vi "M2p_AD_Std_ABA.vi"() -> ()   [LabVIEW 2015]
uses:
  spcm_library/spcm_gui_common.llb/element_device.ctl
  spcm_library/spcm_gui_common.llb/element_mode.ctl
  spcm_library/spcm_gui_m2p.llb/element_m2p_ai_channel.ctl
  spcm_library/spcm_gui_common.llb/element_device_infos.ctl
  spcm_library/spcm_gui_m2p.llb/element_m2p_clock.ctl
  spcm_library/spcm_gui_m2p.llb/element_m2p_ai_trigger.ctl
panel:
  in  "Trigger Settings":T1={"Trigger Source"=0, "External Trigger"=0, "Level 0 Ext"=1500, "Ext Trig Term"=FALSE, "Channel Trigger"=0, "Level 0 Ch"=0, "Level 1 Ch"=0, "Trigger Delay (Samples)"=0} {"Channel Trigger" items=["None", "Pos. Edge", "Neg. Edge", "Any Edge", "Pos. Rearm", "Neg. Rearm", "Enter Window", "Leave Window", "In Win", "Out Win"]; "External Trigger" items=["None", "Pos. Edge", "Neg. Edge", "Any Edge", "High Level", "Low Level"]; "Trigger Source" items=["Software Trigger", "External Trigger", "Channel 0 Trigger", "Channel 1 Trigger", "Channel 2 Trigger", "Channel 3 Trigger", "Channel 4 Trigger", "Channel 5 Trigger", "Channel 6 Trigger", "Channel 7 Trigger"]; "Trigger Delay (Samples)" max=65535 step=1}
  in  "Clock Settings":T2={"Clock Mode"=0, "Sampling Rate (kHz)"=10000.0, "Clock Output"=FALSE, "Termination"=FALSE, "Ref. Clock (MHz)"=10.0, "Threshold (mV)"=1500} {"Threshold (mV)" min=-5000 max=5000; "Clock Mode" items=["Internal Clock Quartz", "External Clock", "External Reference Clock"]; "Ref. Clock (MHz)" min=0.0 max=125000.0; "Sampling Rate (kHz)" min=1.0 max=5000000.0}
  out "Device Infos":T3={"Device Name"="M2p.5942-x4", "Serial Number"=666.0, "Mem (MB)"=1024.0}
  in  "AI Channel 7":T4={"Enable"=TRUE, "Input Range "=2, "Termination"=0, "Input Type"=0, "Offset"=0} {"Input Type" items=["Single-ended", "Differential"]; "Termination" items=["1 MOhm", "50 Ohm"]; "Input Range" items=["±200 mV", "±500 mV", "±1000 mV", "±2000 mV", "±5000 mV", "±10000 mV"]}
  in  "AI Channel 6":T4={"Enable"=TRUE, "Input Range "=2, "Termination"=0, "Input Type"=0, "Offset"=0} {"Input Type" items=["Single-ended", "Differential"]; "Termination" items=["1 MOhm", "50 Ohm"]; "Input Range" items=["±200 mV", "±500 mV", "±1000 mV", "±2000 mV", "±5000 mV", "±10000 mV"]}
  in  "AI Channel 5":T4={"Enable"=TRUE, "Input Range "=2, "Termination"=0, "Input Type"=0, "Offset"=0} {"Input Type" items=["Single-ended", "Differential"]; "Termination" items=["1 MOhm", "50 Ohm"]; "Input Range" items=["±200 mV", "±500 mV", "±1000 mV", "±2000 mV", "±5000 mV", "±10000 mV"]}
  in  "AI Channel 4":T4={"Enable"=TRUE, "Input Range "=2, "Termination"=0, "Input Type"=0, "Offset"=0} {"Input Type" items=["Single-ended", "Differential"]; "Termination" items=["1 MOhm", "50 Ohm"]; "Input Range" items=["±200 mV", "±500 mV", "±1000 mV", "±2000 mV", "±5000 mV", "±10000 mV"]}
  in  "AI Channel 3":T4={"Enable"=TRUE, "Input Range "=2, "Termination"=0, "Input Type"=0, "Offset"=0} {"Input Type" items=["Single-ended", "Differential"]; "Termination" items=["1 MOhm", "50 Ohm"]; "Input Range" items=["±200 mV", "±500 mV", "±1000 mV", "±2000 mV", "±5000 mV", "±10000 mV"]}
  in  "AI Channel 2":T4={"Enable"=TRUE, "Input Range "=2, "Termination"=0, "Input Type"=0, "Offset"=0} {"Input Type" items=["Single-ended", "Differential"]; "Termination" items=["1 MOhm", "50 Ohm"]; "Input Range" items=["±200 mV", "±500 mV", "±1000 mV", "±2000 mV", "±5000 mV", "±10000 mV"]}
  in  "AI Channel 1":T4={"Enable"=TRUE, "Input Range "=2, "Termination"=0, "Input Type"=0, "Offset"=0} {"Input Type" items=["Single-ended", "Differential"]; "Termination" items=["1 MOhm", "50 Ohm"]; "Input Range" items=["±200 mV", "±500 mV", "±1000 mV", "±2000 mV", "±5000 mV", "±10000 mV"]}
  in  "AI Channel 0":T4={"Enable"=TRUE, "Input Range "=2, "Termination"=0, "Input Type"=0, "Offset"=0} {"Input Type" items=["Single-ended", "Differential"]; "Termination" items=["1 MOhm", "50 Ohm"]; "Input Range" items=["±200 mV", "±500 mV", "±1000 mV", "±2000 mV", "±5000 mV", "±10000 mV"]}
  in  "Mode Setup":T5={"Mode"=3, "Mem"=16384, "Seg"=4096, "Post"=4000, "Pre"=32, "ABA"=1024} {"Mode" items=["Singleshot", "Multiple Recording", "Gated Sampling", "ABA Mode"]; "ABA" min=2 max=65535 step=1; "Post" min=4 step=4; "Mem" min=8 step=4; "Pre" min=4 max=8176 step=4; "Seg" min=8 step=4}
  in  "Loop Button":bool
  in  "Singleshot Button":bool
  in  "Quit Button":bool
  in  "Force Trigger Button":bool
  in  "Stop Button":bool
  out "Display ABA Data":sgl[][](graph)=[[-0.7367859, -0.9946289, -0.85287476, -0.3730774, 0.25793457, 0.7870178, 0.54119873, 0.93759155, 0.95895386, 0.5987854, -0.002960205, -0.6014404, -0.95977783, -0.9349365, -0.5342407, 0.078125, 0.6602783, 0.97946167, 0.9064636, 0.47125244, -0.15322876, -0.7137146, -0.9917908, -0.87109375, -0.40386963, 0.22634888, 0.76467896, 0.99749756, 0.8317261, 0.33291626, -0.29797363, -0.80978394, -0.9989319, -0.78674316, -0.262146, 0.36953735, 0.8530884, 0.99542236, 0.957428, 0.9367676, 0.95092773, 0.57244873, 0.9633179, 0.60528564, 0.6083679, 0.96325684, 0.9303894, 0.5276489, -0.08602905, -0.66571045, -0.9791565, -0.90148926, -0.4619751, 0.16055298, 0.7215271, 0.99157715, 0.8659668, 0.39404297, -0.23522949, -0.7704468, -0.9981079, -0.8261719, -0.32208252, 0.3079834, 0.8153076, 0.99713135, 0.7798767, 0.25057983, -0.3774109, -0.8551941, -0.9929199, -0.7310486, -0.17828369, 0.44638062, 0.8932495, 0.9847717, 0.6784668, 0.10494995, -0.51187134, -0.9230957, -0.9657898, -0.6234741, -0.028564453, 0.57696533, 0.9515686, 0.9458008, 0.56240845, -0.046081543, -0.63442993, -0.96972656, -0.9168701, -0.4967041, 0.122802734, 0.69241333, 0.9868469, 0.8860779, 0.43188477, -0.19503784, -0.7442627, -0.99487305, -0.84695435, -0.36273193, 0.26776123, 0.7922363, 0.999115, 0.8059082, 0.29092407, -0.33917236, -0.8347473, -0.99557495, -0.7579651, -0.21740723, 0.41140747, 0.87564087, 0.98968506, 0.70910645, 0.14578247, -0.47720337, -0.908844, -0.9749756, -0.6528015, -0.07043457, 0.5432129, 0.9382324, 0.9571533, 0.5940857, -0.0053100586, -0.60305786, -0.9604492, -0.9328613, -0.53204346, 0.081451416, 0.6625061, 0.9809265, 0.9046936, 0.46777344, -0.15338135, -0.7159729, -0.98999023, -0.86886597, -0.39935303, 0.22888184, 0.76641846, 0.99798584, 0.82928467, 0.32977295, -0.30187988, -0.8128662, -0.9975586, -0.7854004, -0.25775146, 0.37252808, 0.8534241, 0.9945984, 0.73779297, 0.18582153, -0.43966675, -0.88900757, -0.9826355, -0.6835327, -0.109191895, 0.50805664, 0.92178345, 0.96847534, 0.6272888, 0.03527832, -0.56951904, -0.9475403, -0.94628906, -0.56573486, 0.040740967, 0.63171387, 0.96813965, 0.9185791, 0.5029602, -0.11489868, -0.6854553, -0.9836731, -0.8875427, -0.4373169, 0.18899536, 0.7409973, 0.9963074, 0.85150146, 0.36868286, -0.26104736, -0.7892151, -0.99658203, -0.8095093, -0.2960205, 0.33428955, 0.8327942, 0.9961853, 0.76327515, 0.2255249, -0.40457153, -0.869751, -0.9884033, -0.71221924, -0.14993286, 0.47149658, 0.9060974, 0.9775696, 0.65753174, 0.077545166, -0.53515625, -0.9313965, -0.9560852, -0.60009766, -0.0017700195, 0.5982666, 0.9598999, 0.93588257, 0.5386658, -0.07458496, -0.65734863, -0.97714233, -0.9057312, -0.47232056, 0.14935303, 0.71273804, 0.9902649, 0.8724365, 0.40701294, -0.22207642, -0.7612915, -0.99557495, -0.8312683, -0.33428955, 0.2972412, 0.8088684, 0.9990845, 0.78948975, 0.26516724, -0.36514282, -0.8491211, -0.99346924, -0.7403259, -0.1906128, 0.4362793, 0.8887634, 0.9863281, 0.6897888, 0.11758423, -0.5010681, -0.9182129, -0.9694824, -0.6303711, -0.03970337, 0.56658936, 0.94696045, 0.9506836, 0.5725403, -0.032989502, -0.62384033, -0.96728516, -0.9217529, -0.50735474, 0.109802246, 0.6842346, 0.98431396, 0.89172363, 0.4421997, -0.18322754, -0.7343445, -0.99264526, -0.852478, -0.37271118, 0.25668335, 0.78564453, 0.99835205, 0.8143921, 0.3052063, -0.32714844, -0.82696533, -0.9963989, -0.7660217, -0.23092651, 0.3985901, 0.87039185, 0.99102783, 0.71658325, 0.15756226, -0.46670532, -0.9020996, -0.97735596, -0.6616821, -0.081970215, 0.53253174, 0.93270874, 0.96157837, 0.6053772, 0.0068359375, -0.59298706, -0.95565796, -0.936615, -0.5405884, 0.069732666, 0.65304565, 0.97595215, 0.9082947, 0.47894287, -0.14233398, -0.7063904, -0.9873657, -0.87454224, -0.41030884, 0.21688843, 0.7576294, 0.9977722, 0.8375244, 0.34188843, -0.2893982, -0.80496216, -0.99783325, -0.79125977, -0.2698059, 0.36218262, 0.8475952, 0.9964905, 0.7446289, 0.19586182, -0.42956543, -0.8841858, -0.9846802, -0.6915283, -0.12136841, 0.4963379, 0.9172058, 0.97128296, 0.63687134, 0.047454834, -0.56066895, -0.94454956, -0.94888306, -0.5776062, 0.029296875, 0.6207886, 0.9685974, 0.92419434, 0.5151367, -0.10394287, -0.67752075, -0.9823303, -0.8944092, -0.44708252, 0.17849731, 0.73184204, 0.9949646, 0.85809326, 0.3807068, -0.2501526, -0.7796631, -0.99731445, -0.8144226, -0.30908203, 0.32418823, 0.82598877, 0.9975891, 0.77267456, 0.23815918, -0.39318848, -0.86398315, -0.99017334, -0.72213745, -0.16357422, 0.4606018, 0.899353, 0.98202515, 0.6680908, 0.08944702, -0.5254822, -0.93099976, -0.9614258, -0.6101074, -0.013427734, 0.5890198, 0.9560852, 0.9404907, 0.5488281, -0.061035156, -0.6477356, -0.9737854, -0.91049194, -0.48309326, 0.13729858, 0.7044678, 0.9884033, 0.8786316, 0.41744995, -0.21096802, -0.7532959, -0.9957886, -0.8402405, -0.34680176, 0.28399658, 0.8029785, 0.999115, 0.7972717, 0.27694702, -0.35458374, -0.8433533, -0.9954834, -0.74780273, -0.20275879, 0.4248047, 0.88275146, 0.9875488, 0.69647217, 0.12808228, -0.49005127, -0.91326904, -0.9727478, -0.6412964, -0.052947998, 0.55615234, 0.9421997, 0.9526062, 0.58340454, -0.021606445, -0.6161804, -0.9637146, -0.9266052, -0.5185547, 0.097351074, 0.6750183, 0.98391724, 0.89624023, 0.45333862, -0.17086792, -0.727478, -0.9911194, -0.85980225, -0.38391113, 0.2453003, 0.7779846, 0.9977417, 0.8199463, 0.31497192, -0.31588745, -0.82162476, -0.9985962, -0.7744751, -0.24353027, 0.3881836, 0.8618164, 0.99365234, 0.7267761, 0.16906738, -0.45483398, -0.89715576, -0.9794922, -0.6708069, -0.094573975, 0.52267456, 0.9289856, 0.96435547, 0.61550903, 0.019927979, -0.5828247, -0.9527588, -0.94137573, -0.55200195, 0.057128906, 0.6442871, 0.97320557, 0.9138794, 0.48950195, -0.13064575, -0.69818115, -0.98669434, -0.88131714, -0.4220581, 0.20544434, 0.7498779, 0.9970703, 0.8441467, 0.35308838, -0.27630615, -0.7956543, -0.9975891, -0.7987366, -0.2817688, 0.3501892, 0.842926, 0.9965515, 0.75305176, 0.20935059, -0.41931152, -0.87841797, -0.9868164, -0.70007324, -0.13421631, 0.4862671, 0.9122009, 0.9748535, 0.6463318, 0.061462402, -0.5491638, -0.940155, -0.9536133, -0.58636475, 0.015380859, 0.61190796, 0.9640808, 0.9303589, 0.5248413, -0.089416504, -0.6679077, -0.9793701, -0.89849854, -0.45965576], [0.38497925, 0.38497925, 0.38497925, 0.38497925, 0.38497925, 0.38497925, 0.38497925, 0.38497925, 0.38497925, 0.38497925, 0.38497925, 0.38497925, 0.38497925, 0.38497925, 0.38497925, 0.38497925, 0.38497925, 0.38497925, 0.38497925, 0.38497925, 0.38497925, 0.38497925, 0.38497925, 0.38497925, 0.38497925, 0.38497925, 0.38497925, 0.38497925, 0.38497925, 0.38497925, 0.38497925, 0.38497925, 0.38497925, 0.38497925, 0.38497925, 0.38497925, 0.38497925, 0.38497925, 0.38497925, 0.38497925, 0.38497925, 0.38497925, 0.38497925, 0.38497925, 0.38497925, 0.38497925, 0.38497925, 0.38497925, 0.38497925, 0.38497925, 0.38497925, 0.38497925, 0.38497925, 0.38497925, 0.38497925, 0.38497925, 0.38497925, 0.38497925, 0.38497925, 0.38497925, 0.38497925, 0.38497925, 0.38497925, 0.38497925, 0.38497925, 0.38497925, 0.38497925, 0.38497925, 0.38497925, 0.38497925, 0.38497925, 0.38497925, 0.38497925, 0.38497925, 0.38497925, 0.38497925, 0.38497925, 0.38497925, 0.38497925, 0.38497925, 0.38497925, 0.38497925, 0.38497925, 0.38497925, 0.38497925, 0.38497925, 0.38497925, 0.38497925, 0.38497925, 0.38497925, 0.38497925, 0.38497925, 0.38497925, 0.38497925, 0.38497925, 0.38497925, 0.38497925, 0.38497925, 0.38497925, 0.38497925, 0.38497925, 0.38497925, 0.38497925, 0.38497925, 0.38497925, 0.38497925, 0.38497925, 0.38497925, 0.38497925, 0.38497925, 0.38497925, 0.38497925, 0.38497925, 0.38497925, 0.38497925, 0.38497925, 0.38497925, 0.38497925, 0.38497925, 0.38497925, 0.38497925, 0.38497925, 0.38497925, 0.38497925, 0.38497925, 0.38497925, 0.38497925, 0.38497925, 0.38497925, 0.38497925, 0.38497925, 0.38497925, 0.38497925, 0.38497925, 0.38497925, 0.38497925, 0.38497925, 0.38497925, 0.38497925, 0.38497925, 0.38497925, 0.38497925, 0.38497925, 0.38497925, 0.38497925, 0.38497925, 0.38497925, 0.38497925, 0.38497925, 0.38497925, 0.38497925, 0.38497925, 0.38497925, 0.38497925, 0.38497925, 0.38497925, 0.38497925, 0.38497925, 0.38497925, 0.38497925, 0.38497925, 0.38497925, 0.38497925, 0.38497925, 0.38497925, 0.38497925, 0.38497925, 0.38497925, 0.38497925, 0.38497925, 0.38497925, 0.38497925, 0.38497925, 0.38497925, 0.38497925, 0.38497925, 0.38497925, 0.38497925, 0.38497925, 0.38497925, 0.38497925, 0.38497925, 0.38497925, 0.38497925, 0.38497925, 0.38497925, 0.38497925, 0.38497925, 0.38497925, 0.38497925, 0.38497925, 0.38497925, 0.38497925, 0.38497925, 0.38497925, 0.38497925, 0.38497925, 0.38497925, 0.38497925, 0.38497925, 0.38497925, 0.38497925, 0.38497925, 0.38497925, 0.38497925, 0.38497925, 0.38497925, 0.38497925, 0.38497925, 0.38497925, 0.38497925, 0.38497925, 0.38497925, 0.38497925, 0.38497925, 0.38497925, 0.38497925, 0.38497925, 0.38497925, 0.38497925, 0.38497925, 0.38497925, 0.38497925, 0.38497925, 0.38497925, 0.38497925, 0.38497925, 0.38497925, 0.38497925, 0.38497925, 0.38497925, 0.38497925, 0.38497925, 0.38497925, 0.38497925, 0.38497925, 0.38497925, 0.38497925, 0.38497925, 0.38497925, 0.38497925, 0.38497925, 0.38497925, 0.38497925, 0.38497925, 0.38497925, 0.38497925, 0.38497925, 0.38497925, 0.38497925, 0.38497925, 0.38497925, 0.38497925, 0.38497925, 0.38497925, 0.38497925, 0.38497925, 0.38497925, 0.38497925, 0.38497925, 0.38497925, 0.38497925, 0.38497925, 0.38497925, 0.38497925, 0.38497925, 0.38497925, 0.38497925, 0.38497925, 0.38497925, 0.38497925, 0.38497925, 0.38497925, 0.38497925, 0.38497925, 0.38497925, 0.38497925, 0.38497925, 0.38497925, 0.38497925, 0.38497925, 0.38497925, 0.38497925, 0.38497925, 0.38497925, 0.38497925, 0.38497925, 0.38497925, 0.38497925, 0.38497925, 0.38497925, 0.38497925, 0.38497925, 0.38497925, 0.38497925, 0.38497925, 0.38497925, 0.38497925, 0.38497925, 0.38497925, 0.38497925, 0.38497925, 0.38497925, 0.38497925, 0.38497925, 0.38497925, 0.38497925, 0.38497925, 0.38497925, 0.38497925, 0.38497925, 0.38497925, 0.38497925, 0.38497925, 0.38497925, 0.38497925, 0.38497925, 0.38497925, 0.38497925, 0.38497925, 0.38497925, 0.38497925, 0.38497925, 0.38497925, 0.38497925, 0.38497925, 0.38497925, 0.38497925, 0.38497925, 0.38497925, 0.38497925, 0.38497925, 0.38497925, 0.38497925, 0.38497925, 0.38497925, 0.38497925, 0.38497925, 0.38497925, 0.38497925, 0.38497925, 0.38497925, 0.38497925, 0.38497925, 0.38497925, 0.38497925, 0.38497925, 0.38497925, 0.38497925, 0.38497925, 0.38497925, 0.38497925, 0.38497925, 0.38497925, 0.38497925, 0.38497925, 0.38497925, 0.38497925, 0.38497925, 0.38497925, 0.38497925, 0.38497925, 0.38497925, 0.38497925, 0.38497925, 0.38497925, 0.38497925, 0.38497925, 0.38497925, 0.38497925, 0.38497925, 0.38497925, 0.38497925, 0.38497925, 0.38497925, 0.38497925, 0.38497925, 0.38497925, 0.38497925, 0.38497925, 0.38497925, 0.38497925, 0.38497925, 0.38497925, 0.38497925, 0.38497925, 0.38497925, 0.38497925, 0.38497925, 0.38497925, 0.38497925, 0.38497925, 0.38497925, 0.38497925, 0.38497925, 0.38497925, 0.38497925, 0.38497925, 0.38497925, 0.38497925, 0.38497925, 0.38497925, 0.38497925, 0.38497925, 0.38497925, 0.38497925, 0.38497925, 0.38497925, 0.38497925, 0.38497925, 0.38497925, 0.38497925, 0.38497925, 0.38497925, 0.38497925, 0.38497925, 0.38497925, 0.38497925, 0.38497925, 0.38497925, 0.38497925, 0.38497925, 0.38497925, 0.38497925, 0.38497925, 0.38497925, 0.38497925, 0.38497925, 0.38497925, 0.38497925, 0.38497925, 0.38497925, 0.38497925, 0.38497925, 0.38497925, 0.38497925, 0.38497925, 0.38497925, 0.38497925, 0.38497925, 0.38497925, 0.38497925, 0.38497925, 0.38497925, 0.38497925, 0.38497925, 0.38497925, 0.38497925, 0.38497925, 0.38497925, 0.38497925, 0.38497925, 0.38497925, 0.38497925, 0.38497925, 0.38497925, 0.38497925, 0.38497925, 0.38497925, 0.38497925, 0.38497925, 0.38497925, 0.38497925, 0.38497925, 0.38497925, 0.38497925, 0.38497925, 0.38497925, 0.38497925, 0.38497925, 0.38497925, 0.38497925, 0.38497925, 0.38497925, 0.38497925, 0.38497925, 0.38497925, 0.38497925, 0.38497925, 0.38497925, 0.38497925, 0.38497925, 0.38497925, 0.38497925, 0.38497925, 0.38497925, 0.38497925, 0.38497925, 0.38497925, 0.38497925, 0.38497925, 0.38497925, 0.38497925, 0.38497925, 0.38497925, 0.38497925, 0.38497925, 0.38497925, 0.38497925, 0.38497925, 0.38497925, 0.38497925, 0.38497925, 0.38497925, 0.38497925, 0.38497925, 0.38497925, 0.38497925, 0.38497925, 0.38497925, 0.38497925, 0.38497925], [-0.00012207031, -0.00012207031, -6.1035156e-05, -0.00012207031, 0.00015258789, -9.1552734e-05, 0.0, 0.00015258789, -0.00018310547, -6.1035156e-05, -0.00012207031, -3.0517578e-05, 0.00015258789, -0.00012207031, 6.1035156e-05, -3.0517578e-05, -6.1035156e-05, -0.00012207031, -0.00015258789, 0.00012207031, 6.1035156e-05, 3.0517578e-05, 3.0517578e-05, -6.1035156e-05, -0.00012207031, 0.0, 0.0, -6.1035156e-05, -9.1552734e-05, -0.00030517578, 0.0, 0.00015258789, 0.00015258789, -0.00030517578, -0.00015258789, 3.0517578e-05, 0.00018310547, -0.00018310547, -6.1035156e-05, -0.00012207031, -0.00012207031, -9.1552734e-05, -0.00015258789, -6.1035156e-05, -3.0517578e-05, -6.1035156e-05, -6.1035156e-05, -0.0002746582, 0.0, -6.1035156e-05, 3.0517578e-05, 9.1552734e-05, -0.00012207031, 3.0517578e-05, -9.1552734e-05, -9.1552734e-05, 0.00012207031, -3.0517578e-05, -0.00021362305, -6.1035156e-05, 3.0517578e-05, -3.0517578e-05, -6.1035156e-05, 0.0, -9.1552734e-05, 0.00012207031, -0.00018310547, -6.1035156e-05, 3.0517578e-05, 0.00012207031, 0.0002746582, 0.0, -0.00030517578, -0.00039672852, -0.00018310547, 3.0517578e-05, -0.00015258789, 0.00012207031, -0.00012207031, 0.00015258789, 6.1035156e-05, -0.00018310547, -0.00012207031, 0.00015258789, -0.00015258789, 3.0517578e-05, -6.1035156e-05, -0.00012207031, 0.0, 3.0517578e-05, 9.1552734e-05, -3.0517578e-05, -0.00021362305, 6.1035156e-05, -0.00012207031, -0.00018310547, 0.0, 6.1035156e-05, -9.1552734e-05, -0.00018310547, 0.0, -0.00015258789, -0.00021362305, -0.00018310547, 0.00012207031, 6.1035156e-05, 6.1035156e-05, -9.1552734e-05, -6.1035156e-05, -9.1552734e-05, -0.00012207031, 0.00015258789, 6.1035156e-05, 6.1035156e-05, 0.00018310547, -0.00030517578, -3.0517578e-05, 0.00012207031, -9.1552734e-05, -6.1035156e-05, 0.0, -6.1035156e-05, 0.0, -6.1035156e-05, -0.00012207031, 6.1035156e-05, 0.00015258789, 0.00021362305, -0.00015258789, -0.00012207031, -0.00012207031, -0.00012207031, 0.0, -3.0517578e-05, -0.00012207031, 0.0, -6.1035156e-05, 0.00015258789, 0.0, 0.0, 0.0, -9.1552734e-05, 6.1035156e-05, -9.1552734e-05, -3.0517578e-05, 6.1035156e-05, 3.0517578e-05, 3.0517578e-05, -0.00018310547, -0.00018310547, 6.1035156e-05, 0.0, -0.00018310547, -0.0002746582, 0.00012207031, 0.00012207031, -0.0002746582, 9.1552734e-05, 0.0, 9.1552734e-05, -0.00015258789, 6.1035156e-05, -0.0002746582, 0.0, 0.00024414062, 6.1035156e-05, -0.00021362305, -0.00015258789, -0.00021362305, 3.0517578e-05, 0.0, -0.00015258789, 6.1035156e-05, -3.0517578e-05, 0.0, 0.0, 3.0517578e-05, 6.1035156e-05, -0.00018310547, 0.00015258789, 6.1035156e-05, -3.0517578e-05, 3.0517578e-05, -3.0517578e-05, 0.00012207031, 0.00024414062, -6.1035156e-05, -0.00015258789, 0.0, 0.0, -0.00021362305, 9.1552734e-05, -0.00018310547, 6.1035156e-05, 6.1035156e-05, 9.1552734e-05, -6.1035156e-05, -0.00021362305, -0.00021362305, -0.00012207031, -9.1552734e-05, -0.0005187988, 0.00012207031, 0.0, 0.00018310547, 0.0, 0.00018310547, -3.0517578e-05, 0.0, 0.0, -0.00012207031, -6.1035156e-05, -3.0517578e-05, -9.1552734e-05, 9.1552734e-05, -6.1035156e-05, 0.0, 0.00012207031, -3.0517578e-05, -9.1552734e-05, 6.1035156e-05, -0.00018310547, -0.00024414062, -0.00018310547, -6.1035156e-05, -3.0517578e-05, 0.0, 3.0517578e-05, 6.1035156e-05, -9.1552734e-05, -6.1035156e-05, -0.00021362305, 3.0517578e-05, -0.00012207031, 6.1035156e-05, -0.00012207031, 3.0517578e-05, 0.00018310547, 3.0517578e-05, -9.1552734e-05, -9.1552734e-05, -0.00018310547, 0.0, -3.0517578e-05, -6.1035156e-05, -0.00012207031, 9.1552734e-05, 0.0, -0.00012207031, -3.0517578e-05, 3.0517578e-05, 0.00015258789, 0.00021362305, -0.00048828125, -3.0517578e-05, -6.1035156e-05, -0.00012207031, -9.1552734e-05, -6.1035156e-05, -0.00015258789, 0.0, -0.00012207031, 0.00018310547, 0.00012207031, 0.0, 3.0517578e-05, -6.1035156e-05, 9.1552734e-05, 0.00012207031, 6.1035156e-05, -0.00012207031, 6.1035156e-05, 3.0517578e-05, 0.00021362305, -0.00015258789, -6.1035156e-05, 6.1035156e-05, 3.0517578e-05, 0.0, 3.0517578e-05, -3.0517578e-05, 6.1035156e-05, 6.1035156e-05, 0.00012207031, 0.0, 9.1552734e-05, 3.0517578e-05, -0.00018310547, -0.00012207031, 6.1035156e-05, 0.0, -6.1035156e-05, 9.1552734e-05, -6.1035156e-05, 0.0, -6.1035156e-05, 0.0, -9.1552734e-05, 3.0517578e-05, 6.1035156e-05, -6.1035156e-05, -0.00015258789, -0.00012207031, 0.0, -9.1552734e-05, -0.00018310547, -6.1035156e-05, -0.00012207031, 3.0517578e-05, 0.00018310547, -0.00012207031, 9.1552734e-05, 0.00015258789, 0.00018310547, -0.00015258789, 6.1035156e-05, -0.00024414062, -0.00012207031, 0.00015258789, -0.00021362305, 0.0, 0.0, 0.00024414062, 6.1035156e-05, 0.0, 3.0517578e-05, 0.0, -0.00015258789, -9.1552734e-05, 0.00012207031, -3.0517578e-05, 6.1035156e-05, -0.00021362305, -9.1552734e-05, -3.0517578e-05, 6.1035156e-05, -0.00015258789, -6.1035156e-05, -0.00021362305, -3.0517578e-05, 9.1552734e-05, -3.0517578e-05, -0.00015258789, 0.0, 0.0, 0.0, -9.1552734e-05, 0.00012207031, -0.00018310547, -0.00024414062, -0.00021362305, 0.00012207031, -0.00015258789, -9.1552734e-05, -0.00024414062, -3.0517578e-05, 0.0, 0.00033569336, 0.0, -0.00021362305, 9.1552734e-05, -6.1035156e-05, -0.00021362305, -3.0517578e-05, -0.00012207031, -9.1552734e-05, -0.00036621094, -0.0002746582, -0.00015258789, 6.1035156e-05, -3.0517578e-05, 0.00030517578, 0.0, -0.00012207031, 0.00018310547, -3.0517578e-05, -0.00015258789, -6.1035156e-05, 6.1035156e-05, 0.0, 9.1552734e-05, -0.00015258789, -6.1035156e-05, -0.00015258789, -3.0517578e-05, 0.0, -0.00021362305, -6.1035156e-05, -9.1552734e-05, -3.0517578e-05, 3.0517578e-05, -0.00012207031, -0.0002746582, -3.0517578e-05, 0.00012207031, -0.00012207031, -0.00012207031, -0.00030517578, -0.00021362305, 3.0517578e-05, 0.00012207031, 0.0, 3.0517578e-05, 6.1035156e-05, -9.1552734e-05, -3.0517578e-05, 0.00015258789, 0.00012207031, 3.0517578e-05, 3.0517578e-05, -6.1035156e-05, -0.00015258789, -3.0517578e-05, -3.0517578e-05, -9.1552734e-05, -3.0517578e-05, -6.1035156e-05, -0.00012207031, 0.0, -0.00018310547, 3.0517578e-05, -6.1035156e-05, 0.0, 3.0517578e-05, -3.0517578e-05, -3.0517578e-05, -0.00012207031, 0.0, 6.1035156e-05, -9.1552734e-05, 6.1035156e-05, -0.00015258789, -0.00021362305, -0.00021362305, 3.0517578e-05, -3.0517578e-05, -3.0517578e-05, 6.1035156e-05, -9.1552734e-05, 0.0, -9.1552734e-05, 3.0517578e-05, -0.00015258789, -9.1552734e-05, -3.0517578e-05, -3.0517578e-05, -6.1035156e-05, 0.00015258789, -6.1035156e-05, -0.00021362305, -3.0517578e-05, 9.1552734e-05, -0.00024414062, -3.0517578e-05, -6.1035156e-05, -0.00024414062, 0.0, 9.1552734e-05, -0.00015258789, 6.1035156e-05, -0.00012207031, 0.0, -6.1035156e-05, -0.00012207031, -3.0517578e-05, 0.0, -9.1552734e-05, 9.1552734e-05, -0.00012207031, 9.1552734e-05, -0.0002746582, -0.00012207031, 0.0, 0.00012207031, -3.0517578e-05, 0.0, 0.0, -9.1552734e-05, 9.1552734e-05, -9.1552734e-05, -0.00015258789, 0.0, -0.00018310547, 0.0, -6.1035156e-05, -3.0517578e-05, -3.0517578e-05, 6.1035156e-05, -9.1552734e-05, 9.1552734e-05, -9.1552734e-05, 0.00015258789, -0.00033569336, -3.0517578e-05, 6.1035156e-05, 0.00015258789, 3.0517578e-05, -0.00015258789, 0.00012207031, 9.1552734e-05, 0.0, -9.1552734e-05, -0.00012207031, 0.0, 3.0517578e-05, -9.1552734e-05, -6.1035156e-05, -0.00018310547, -3.0517578e-05, -0.00021362305, 9.1552734e-05, -9.1552734e-05], [0.1260376, 0.1260376, 0.1260376, 0.1260376, 0.1260376, 0.1260376, 0.1260376, 0.1260376, 0.1260376, 0.1260376, 0.1260376, 0.1260376, 0.1260376, 0.1260376, 0.1260376, 0.1260376, 0.1260376, 0.1260376, 0.1260376, 0.1260376, 0.1260376, 0.1260376, 0.1260376, 0.1260376, 0.1260376, 0.1260376, 0.1260376, 0.1260376, 0.1260376, 0.1260376, 0.1260376, 0.1260376, 0.1260376, 0.1260376, 0.1260376, 0.1260376, 0.1260376, 0.1260376, 0.1260376, 0.1260376, 0.1260376, 0.1260376, 0.1260376, 0.1260376, 0.1260376, 0.1260376, 0.1260376, 0.1260376, 0.1260376, 0.1260376, 0.1260376, 0.1260376, 0.1260376, 0.1260376, 0.1260376, 0.1260376, 0.1260376, 0.1260376, 0.1260376, 0.1260376, 0.1260376, 0.1260376, 0.1260376, 0.1260376, 0.1260376, 0.1260376, 0.1260376, 0.1260376, 0.1260376, 0.1260376, 0.1260376, 0.1260376, 0.1260376, 0.1260376, 0.1260376, 0.1260376, 0.1260376, 0.1260376, 0.1260376, 0.1260376, 0.1260376, 0.1260376, 0.1260376, 0.1260376, 0.1260376, 0.1260376, 0.1260376, 0.1260376, 0.1260376, 0.1260376, 0.1260376, 0.1260376, 0.1260376, 0.1260376, 0.1260376, 0.1260376, 0.1260376, 0.1260376, 0.1260376, 0.1260376, 0.1260376, 0.1260376, 0.1260376, 0.1260376, 0.1260376, 0.1260376, 0.1260376, 0.1260376, 0.1260376, 0.1260376, 0.1260376, 0.1260376, 0.1260376, 0.1260376, 0.1260376, 0.1260376, 0.1260376, 0.1260376, 0.1260376, 0.1260376, 0.1260376, 0.1260376, 0.1260376, 0.1260376, 0.1260376, 0.1260376, 0.1260376, 0.1260376, 0.1260376, 0.1260376, 0.1260376, 0.1260376, 0.1260376, 0.1260376, 0.1260376, 0.1260376, 0.1260376, 0.1260376, 0.1260376, 0.1260376, 0.1260376, 0.1260376, 0.1260376, 0.1260376, 0.1260376, 0.1260376, 0.1260376, 0.1260376, 0.1260376, 0.1260376, 0.1260376, 0.1260376, 0.1260376, 0.1260376, 0.1260376, 0.1260376, 0.1260376, 0.1260376, 0.1260376, 0.1260376, 0.1260376, 0.1260376, 0.1260376, 0.1260376, 0.1260376, 0.1260376, 0.1260376, 0.1260376, 0.1260376, 0.1260376, 0.1260376, 0.1260376, 0.1260376, 0.1260376, 0.1260376, 0.1260376, 0.1260376, 0.1260376, 0.1260376, 0.1260376, 0.1260376, 0.1260376, 0.1260376, 0.1260376, 0.1260376, 0.1260376, 0.1260376, 0.1260376, 0.1260376, 0.1260376, 0.1260376, 0.1260376, 0.1260376, 0.1260376, 0.1260376, 0.1260376, 0.1260376, 0.1260376, 0.1260376, 0.1260376, 0.1260376, 0.1260376, 0.1260376, 0.1260376, 0.1260376, 0.1260376, 0.1260376, 0.1260376, 0.1260376, 0.1260376, 0.1260376, 0.1260376, 0.1260376, 0.1260376, 0.1260376, 0.1260376, 0.1260376, 0.1260376, 0.1260376, 0.1260376, 0.1260376, 0.1260376, 0.1260376, 0.1260376, 0.1260376, 0.1260376, 0.1260376, 0.1260376, 0.1260376, 0.1260376, 0.1260376, 0.1260376, 0.1260376, 0.1260376, 0.1260376, 0.1260376, 0.1260376, 0.1260376, 0.1260376, 0.1260376, 0.1260376, 0.1260376, 0.1260376, 0.1260376, 0.1260376, 0.1260376, 0.1260376, 0.1260376, 0.1260376, 0.1260376, 0.1260376, 0.1260376, 0.1260376, 0.1260376, 0.1260376, 0.1260376, 0.1260376, 0.1260376, 0.1260376, 0.1260376, 0.1260376, 0.1260376, 0.1260376, 0.1260376, 0.1260376, 0.1260376, 0.1260376, 0.1260376, 0.1260376, 0.1260376, 0.1260376, 0.1260376, 0.1260376, 0.1260376, 0.1260376, 0.1260376, 0.1260376, 0.1260376, 0.1260376, 0.1260376, 0.1260376, 0.1260376, 0.1260376, 0.1260376, 0.1260376, 0.1260376, 0.1260376, 0.1260376, 0.1260376, 0.1260376, 0.1260376, 0.1260376, 0.1260376, 0.1260376, 0.1260376, 0.1260376, 0.1260376, 0.1260376, 0.1260376, 0.1260376, 0.1260376, 0.1260376, 0.1260376, 0.1260376, 0.1260376, 0.1260376, 0.1260376, 0.1260376, 0.1260376, 0.1260376, 0.1260376, 0.1260376, 0.1260376, 0.1260376, 0.1260376, 0.1260376, 0.1260376, 0.1260376, 0.1260376, 0.1260376, 0.1260376, 0.1260376, 0.1260376, 0.1260376, 0.1260376, 0.1260376, 0.1260376, 0.1260376, 0.1260376, 0.1260376, 0.1260376, 0.1260376, 0.1260376, 0.1260376, 0.1260376, 0.1260376, 0.1260376, 0.1260376, 0.1260376, 0.1260376, 0.1260376, 0.1260376, 0.1260376, 0.1260376, 0.1260376, 0.1260376, 0.1260376, 0.1260376, 0.1260376, 0.1260376, 0.1260376, 0.1260376, 0.1260376, 0.1260376, 0.1260376, 0.1260376, 0.1260376, 0.1260376, 0.1260376, 0.1260376, 0.1260376, 0.1260376, 0.1260376, 0.1260376, 0.1260376, 0.1260376, 0.1260376, 0.1260376, 0.1260376, 0.1260376, 0.1260376, 0.1260376, 0.1260376, 0.1260376, 0.1260376, 0.1260376, 0.1260376, 0.1260376, 0.1260376, 0.1260376, 0.1260376, 0.1260376, 0.1260376, 0.1260376, 0.1260376, 0.1260376, 0.1260376, 0.1260376, 0.1260376, 0.1260376, 0.1260376, 0.1260376, 0.1260376, 0.1260376, 0.1260376, 0.1260376, 0.1260376, 0.1260376, 0.1260376, 0.1260376, 0.1260376, 0.1260376, 0.1260376, 0.1260376, 0.1260376, 0.1260376, 0.1260376, 0.1260376, 0.1260376, 0.1260376, 0.1260376, 0.1260376, 0.1260376, 0.1260376, 0.1260376, 0.1260376, 0.1260376, 0.1260376, 0.1260376, 0.1260376, 0.1260376, 0.1260376, 0.1260376, 0.1260376, 0.1260376, 0.1260376, 0.1260376, 0.1260376, 0.1260376, 0.1260376, 0.1260376, 0.1260376, 0.1260376, 0.1260376, 0.1260376, 0.1260376, 0.1260376, 0.1260376, 0.1260376, 0.1260376, 0.1260376, 0.1260376, 0.1260376, 0.1260376, 0.1260376, 0.1260376, 0.1260376, 0.1260376, 0.1260376, 0.1260376, 0.1260376, 0.1260376, 0.1260376, 0.1260376, 0.1260376, 0.1260376, 0.1260376, 0.1260376, 0.1260376, 0.1260376, 0.1260376, 0.1260376, 0.1260376, 0.1260376, 0.1260376, 0.1260376, 0.1260376, 0.1260376, 0.1260376, 0.1260376, 0.1260376, 0.1260376, 0.1260376, 0.1260376, 0.1260376, 0.1260376, 0.1260376, 0.1260376, 0.1260376, 0.1260376, 0.1260376, 0.1260376, 0.1260376, 0.1260376, 0.1260376, 0.1260376, 0.1260376, 0.1260376, 0.1260376, 0.1260376, 0.1260376, 0.1260376, 0.1260376, 0.1260376, 0.1260376, 0.1260376, 0.1260376, 0.1260376, 0.1260376, 0.1260376, 0.1260376, 0.1260376, 0.1260376, 0.1260376, 0.1260376, 0.1260376, 0.1260376, 0.1260376, 0.1260376, 0.1260376, 0.1260376, 0.1260376]]
  out "Write Setup":bool
  out "Status":string="Stopped"
  out "Display Data":sgl[][](graph)
  in  "Device":T6 {"Device" items=["Card", "digitizerNETBOX"]}
  # "M2p ABA Example"
  # "Mode Settings"
  # "Range"
  # "Term"
  # "Type"
  # "Offset"
  # "Ch0"
  # "Ch1"
  # "Clock Settings"
  # "Ch2"
  # "Ch3"
  # "Ch4"
  # "Trigger Settings"
  # "Ch5"
  # "Ch6"
  # "Ch7"
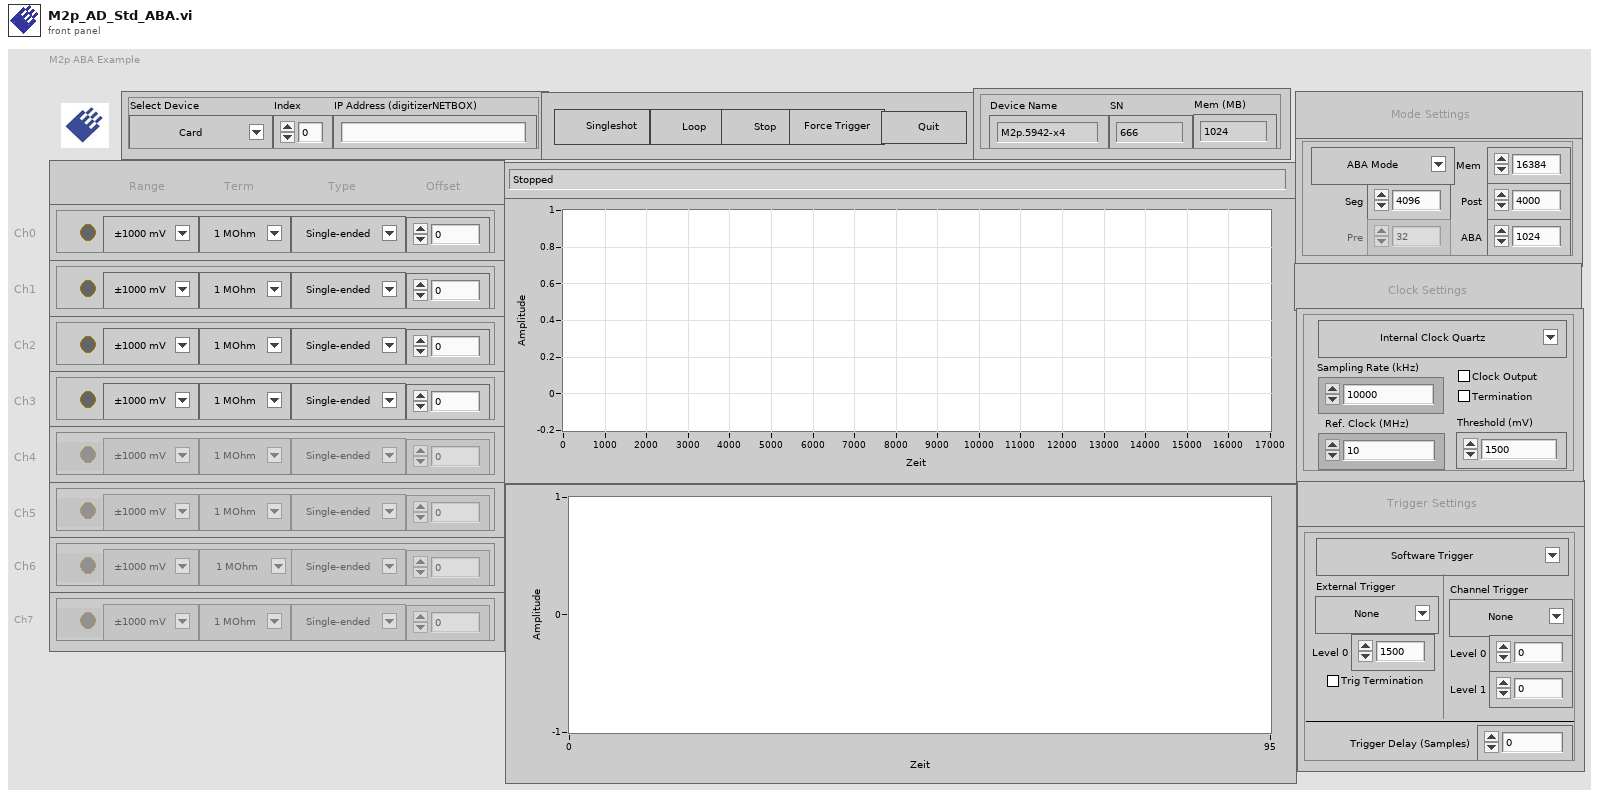
[diagram p1: front panel]
types:
  T1 = typedef "element_m2p_ai_trigger.ctl" = cluster{"Trigger Source":u16, "External Trigger":u16, "Level 0 Ext":i32, "Ext Trig Term":bool, "Channel Trigger":u16, "Level 0 Ch":i32, "Level 1 Ch":i32, "Trigger Delay (Samples)":u32}
  T2 = typedef "element_m2p_clock.ctl" = cluster{"Clock Mode":u16, "Sampling Rate (kHz)":dbl, "Clock Output":bool, "Termination":bool, "Ref. Clock (MHz)":dbl, "Threshold (mV)":i32}
  T3 = typedef "element_device_infos.ctl" = cluster{"Device Name":string, "Serial Number":dbl, "Mem (MB)":dbl}
  T4 = typedef "element_m2p_ai_channel.ctl" = cluster{"Enable":bool, "Input Range ":u16, "Termination":u16, "Input Type":u16, "Offset":i32}
  T5 = typedef "element_mode.ctl" = cluster{"Mode":u16, "Mem":u32, "Seg":u32, "Post":u32, "Pre":u32, "ABA":u32}
  T6 = typedef "element_device.ctl" = cluster{"Index":dbl, "IP Address":string, "Device":u16}
  T7 = enum16{"Idle", "Init", "Write Setup", "Start", "Acquire", "Read Data", "Stop", "Quit"}
  T8 = cluster{"Card Type":i32, "Inst Mem (high part)":i32, "Inst Mem (low part)":i32, "Serial Number":i32, "Function Type":i32, "Installed Features":i32, "Base Card Version":i32, "Module Version":i32, "Extension Version":i32, "Production Date":i32, "Max Sampling Rate":i32, "Max Channels":i32, "Demo Card":i32}
  T9 = cluster{"Card Name":string, "SN":i32, "Mem (MB)":i32}
  T10 = cluster{"AI Channels":i32, "AI Ranges":i32, "Input Ranges (mV)":i32[], "Programmable Offset":i32, "Termination Available":bool, "SE/Diff switchable":bool, "Offset in per cent/mV":bool, "Offset Calibration":bool, "Gain Calibration":bool, "Offset with open inputs":bool, "AI Range Strings[]":string[], "Bit Resolution":i32, "AC Coupling available":bool, "BW Limit available":bool, "AI Path count":i32}
  T11 = enum16{"Idle", "Init", "Write Setup", "Start", "Acquire", "Read Data", "Quit"}
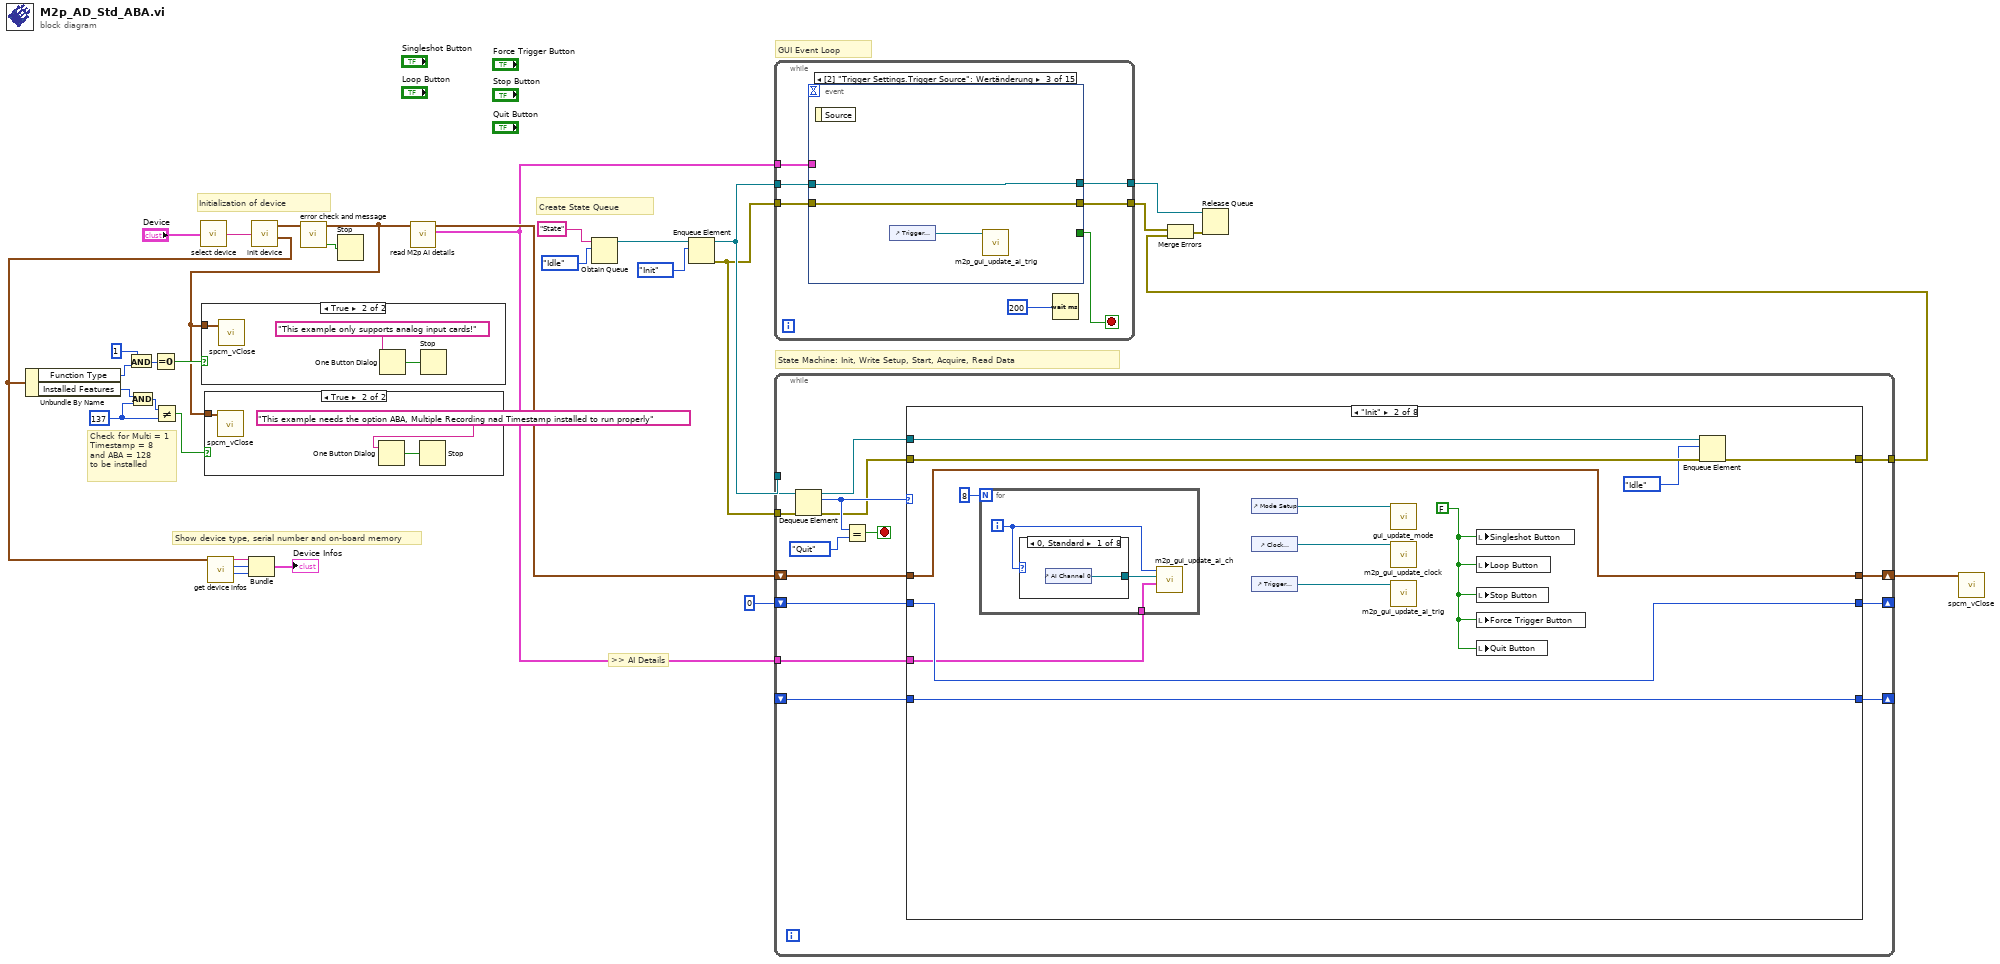
[diagram p0: block diagram]
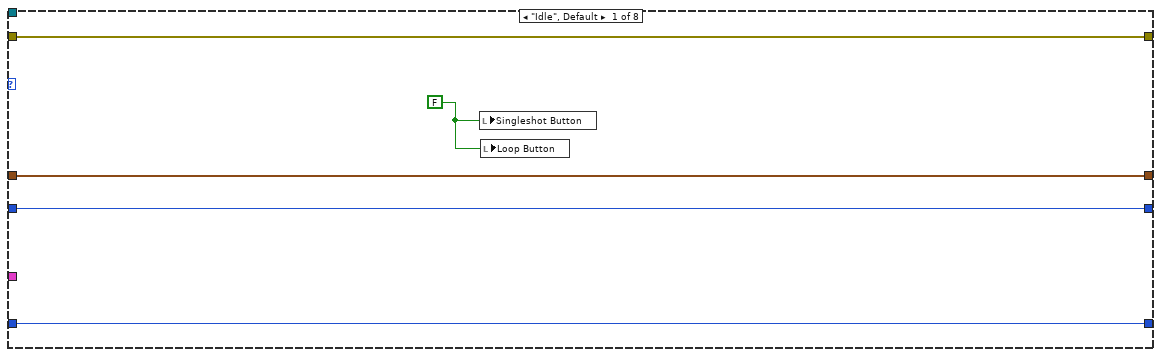
[diagram p4: hidden frame]
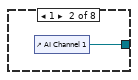
[diagram p5: hidden frame]
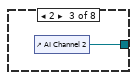
[diagram p6: hidden frame]
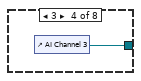
[diagram p7: hidden frame]
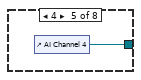
[diagram p8: hidden frame]
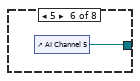
[diagram p9: hidden frame]
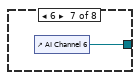
[diagram p10: hidden frame]
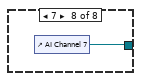
[diagram p11: hidden frame]
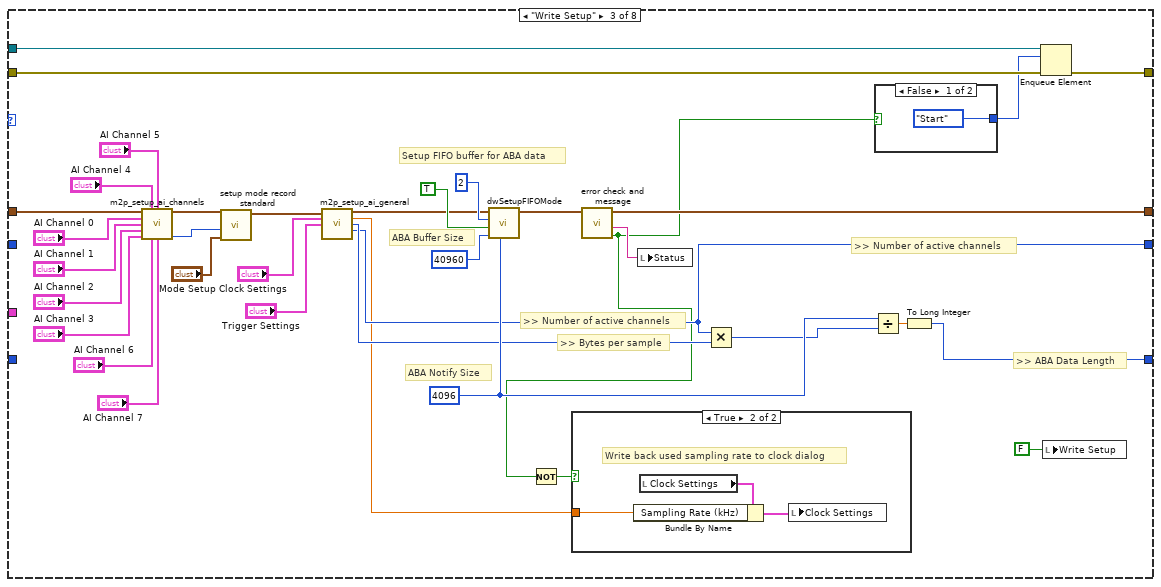
[diagram p12: hidden frame]
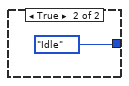
[diagram p14: hidden frame]
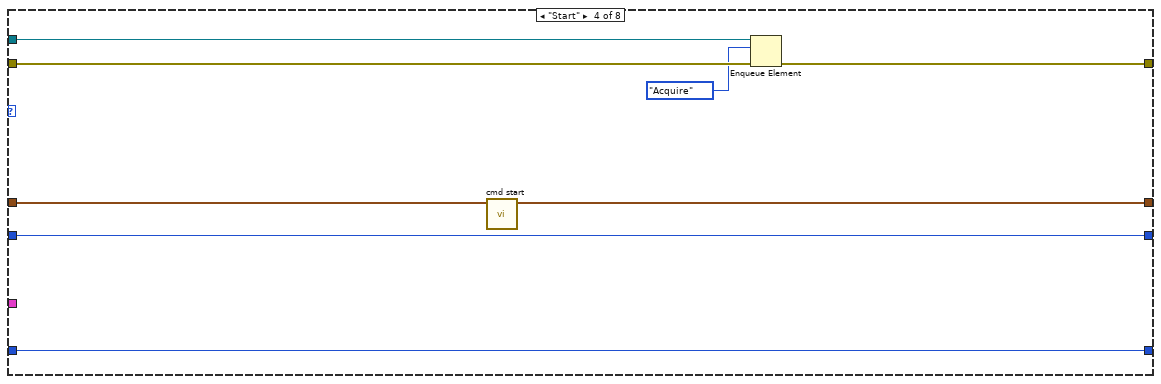
[diagram p15: hidden frame]
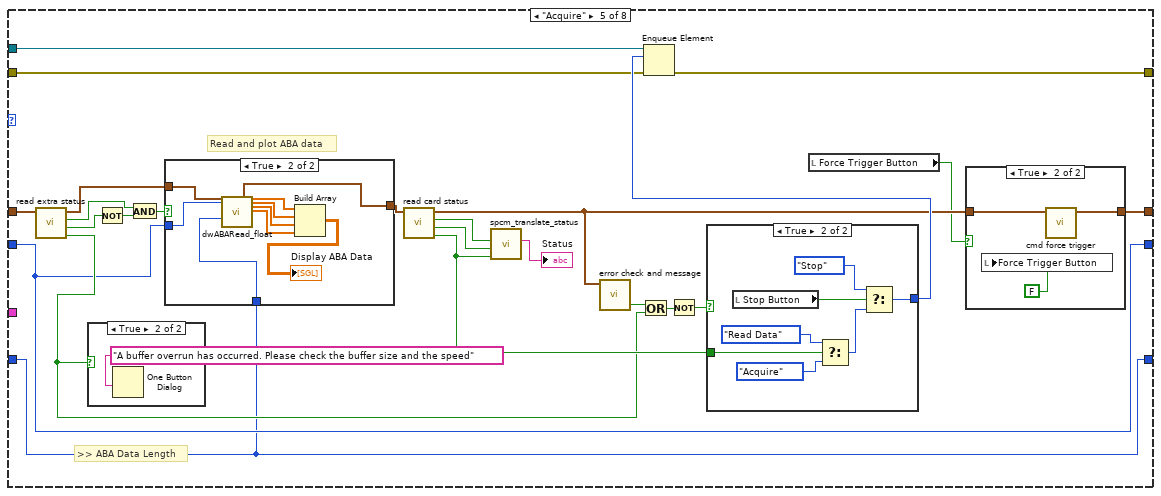
[diagram p16: hidden frame]
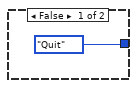
[diagram p19: hidden frame]
diagram:
  w6 = 137
  # "Show device type, serial number and on-board memory"
  # "Check for Multi = 1\nTimestamp = 8\nand ABA = 128\nto be installed"
  # ">> AI Details"
  # "Initialization of device"
  # "Create State Queue"
  # "State Machine: Init, Write Setup, Start, Acquire, Read Data"
  # "GUI Event Loop"
  n1 = call "select device.vi"("Device"="Device") -> ("device string"=w32:string)  [unwired: 4 in]
  n2 = call "init device.vi"("Device String"=w32) -> ("Card Info Out"=w31:cluster{"Card Handle":u64, "Error Code":u32}, "Card Information"=w16:T8)  [unwired: 4 in]
  n3 = Unbundle By Name(w16) -> ("Function Type"=w20:i32, "Installed Features"=w8:i32)
  n4 = And(x=1, y=w20) -> (x .and. y?=w19:i32)
  n5 = And(x=w8, y=w6) -> (x .and. y?=w7:i32)
  n6 = Equal To 0?(x=w19) -> (x = 0?=w17:bool)
  n7 = Not Equal?(x=w7, y=w6) -> (x != y?=w5:bool)
  n8 = call "get device infos.vi"("Card Information"=w16) -> ("Mem (MB)"=w23:i32, "SN"=w22:i32, "Card Name"=w21:string)  [unwired: 8 in]
  n9 = Bundle("Card Name"=w21, "SN"=w22, "Mem (MB)"=w23) -> (→"Device Infos":T9)  [unwired: 1 in]
  n10 = call "error check and message.vi"("Card Info In"=w31) -> ("Error occurred"=w30:bool, "Card Info Out"=w4:cluster{"Card Handle":u64, "Error Code":u32})  [unwired: 4 in, 1 out]
  n11 = case shown="True" w17 {
    tunnel: w4 -> [_ w33]
    frame False {
    }
    frame True {
      n12 = call "spcm_vClose.vi"("Card Info In"=w33) -> ()  [unwired: 7 in]
      n13 = One Button Dialog(message="This example only supports analog input cards!") -> (true=w34:bool)  [unwired: 1 in]
      n14 = Stop(stop? (T)=w34) -> ()
    }
  }
  n15 = case shown="True" w5 {
    tunnel: w4 -> [_ w36]
    frame False {
    }
    frame True {
      n16 = call "spcm_vClose.vi"("Card Info In"=w36) -> ()  [unwired: 7 in]
      n17 = One Button Dialog(message="This example needs the option ABA, Multiple Recording nad Timestamp installed to run properly") -> (true=w38:bool)  [unwired: 1 in]
      n18 = Stop(stop? (T)=w38) -> ()
    }
  }
  n19 = Stop(stop? (T)=w30) -> ()
  n20 = call "read M2p AI details.vi"("Card Info In"=w4) -> ("AI Details"=w2:T10, "Card Info Out"=w3:cluster{"Card Handle":u64, "Error Code":u32})  [unwired: 5 in]
  n21 = Obtain Queue(name (unnamed)="State", element data type=T7."Idle") -> (queue out=w27:refnum<queue>)  [unwired: 3 in, 2 out]
  n22 = Enqueue Element(queue=w27, element=T7."Init") -> (queue out=w28:refnum<queue>, error out=w11:errorcluster)  [unwired: 2 in, 1 out]
  n23 = while {
    tunnel: w28 -> [w43]
    tunnel: [w44] -> w12
    tunnel: [w40] -> w15
    tunnel: w11 -> [w41]
    tunnel: w2 -> [w39]
    stop <- w42 stop-if-true
    n24 = event shown="[2] \"Trigger Settings.Trigger Source\": Wertänderung" {
      selector: _ -> [_ _ _ _ _ _ _ _ _ _ _ _ _ _ _]
      dyn-events: _ -> [_ _ _ _ _ _ _ _ _ _ _ _ _ _ _]
      timeout: _ -> [_ _ _ _ _ _ _ _ _ _ _ _ _ _ _]
      tunnel: [_ _ _ _ _ _ _ _ _ _ _ _ _ TRUE _] -> w42
      tunnel: [w48 w51 w54 w59 w64 w69 w74 w76 w81 _ _ w95 w100 w105 w109] -> w44
      tunnel: w43 -> [w48 w51 w54 w59 w64 w69 w74 w76 w81 _ _ w94 w99 w106 w109]
      tunnel: [w47 w50 w53 w58 w63 w68 w73 w75 w80 _ _ w92 w97 w103 w108] -> w40
      tunnel: w41 -> [w47 w50 w53 w58 w63 w68 w73 w75 w80 _ _ w93 w98 w102 w108]
      tunnel: w39 -> [_ _ _ w55 w60 w65 w70 w77 w82 w85 w88 _ _ _ _]
      event Value Change {
        n25 = event-data ("Ereignisdatenknoten")() -> ()  [unwired: 1 in, 1 out]
        n26 = control-ref of="Mode Setup"() -> (w46:refnum<vi>)
        n27 = call "gui_update_mode.vi"("Referenz Mode Settings"=w46) -> ()  [unwired: 11 in]
      }
      event Value Change {
        n28 = event-data() -> ()  [unwired: 1 in, 1 out]
        n29 = control-ref of="Clock Settings"() -> (w49:refnum<vi>)
        n30 = call "m2p_gui_update_clock.vi"("Cluster Reference"=w49) -> ()  [unwired: 11 in]
      }
      event Value Change {
        n31 = event-data() -> ()  [unwired: 1 in, 1 out]
        n32 = control-ref of="Trigger Settings"() -> (w52:refnum<vi>)
        n33 = call "m2p_gui_update_ai_trig.vi"("Trigger Settings Reference"=w52) -> ()  [unwired: 10 in]
      }
      event Value Change {
        n34 = event-data() -> ()  [unwired: 1 in, 1 out]
        n35 = control-ref of="AI Channel 0"() -> (w56:refnum<vi>)
        n36 = call "m2p_gui_update_ai_ch.vi"("AI Details"=w55, "Cluster Referenz"=w56, "Channel Index"=0) -> ()  [unwired: 9 in]
      }
      event Value Change {
        n37 = event-data() -> ()  [unwired: 1 in, 1 out]
        n38 = control-ref of="AI Channel 1"() -> (w61:refnum<vi>)
        n39 = call "m2p_gui_update_ai_ch.vi"("AI Details"=w60, "Cluster Referenz"=w61, "Channel Index"=1) -> ()  [unwired: 9 in]
      }
      event Value Change {
        n40 = event-data() -> ()  [unwired: 1 in, 1 out]
        n41 = control-ref of="AI Channel 2"() -> (w66:refnum<vi>)
        n42 = call "m2p_gui_update_ai_ch.vi"("AI Details"=w65, "Cluster Referenz"=w66, "Channel Index"=2) -> ()  [unwired: 9 in]
      }
      event Value Change {
        n43 = event-data() -> ()  [unwired: 1 in, 1 out]
        n44 = control-ref of="AI Channel 3"() -> (w71:refnum<vi>)
        n45 = call "m2p_gui_update_ai_ch.vi"("AI Details"=w70, "Cluster Referenz"=w71, "Channel Index"=3) -> ()  [unwired: 9 in]
      }
      event Value Change {
        n46 = event-data() -> ()  [unwired: 1 in, 1 out]
        n47 = control-ref of="AI Channel 4"() -> (w78:refnum<vi>)
        n48 = call "m2p_gui_update_ai_ch.vi"("AI Details"=w77, "Cluster Referenz"=w78, "Channel Index"=4) -> ()  [unwired: 9 in]
      }
      event Value Change {
        n49 = event-data() -> ()  [unwired: 1 in, 1 out]
        n50 = control-ref of="AI Channel 5"() -> (w83:refnum<vi>)
        n51 = call "m2p_gui_update_ai_ch.vi"("AI Details"=w82, "Cluster Referenz"=w83, "Channel Index"=5) -> ()  [unwired: 9 in]
      }
      event Value Change {
        n52 = event-data() -> ()  [unwired: 1 in, 1 out]
        n53 = control-ref of="AI Channel 6"() -> (w86:refnum<vi>)
        n54 = call "m2p_gui_update_ai_ch.vi"("AI Details"=w85, "Cluster Referenz"=w86, "Channel Index"=6) -> ()  [unwired: 9 in]
      }
      event Value Change {
        n55 = event-data() -> ()  [unwired: 1 in, 1 out]
        n56 = control-ref of="AI Channel 7"() -> (w89:refnum<vi>)
        n57 = call "m2p_gui_update_ai_ch.vi"("AI Details"=w88, "Cluster Referenz"=w89, "Channel Index"=7) -> ()  [unwired: 9 in]
      }
      event "Singleshot Button", "Loop Button": Value Change {
        n58 = event-data() -> ()  [unwired: 1 in, 1 out]
        n59 = Enqueue Element(queue=w94, element=T7."Write Setup", error in (no error)=w93) -> (queue out=w95:refnum<queue>, error out=w92:errorcluster)  [unwired: 1 in, 1 out]
      }
      event "Stop Button": Value Change {
        n60 = event-data() -> ()  [unwired: 1 in, 1 out]
        n61 = Enqueue Element(queue=w99, element=T7."Idle", error in (no error)=w98) -> (queue out=w100:refnum<queue>, error out=w97:errorcluster)  [unwired: 1 in, 1 out]
      }
      event "Quit Button": Value Change {
        n62 = event-data() -> ()  [unwired: 1 in, 1 out]
        n63 = Enqueue Element(queue=w106, element=T7."Quit", error in (no error)=w102) -> (queue out=w105:refnum<queue>, error out=w103:errorcluster)  [unwired: 1 in, 1 out]
      }
      event Value Change {
        n64 = event-data() -> ()  [unwired: 1 in, 1 out]
        "Write Setup" <- TRUE
      }
    }
    n65 = Wait (ms)(milliseconds to wait=200) -> ()  [unwired: 1 out]
  }
  n66 = while {
    tunnel: w28 -> [w124]
    shift-right: [w122] -> w26
    shift-left: w3 -> [w123]
    shift-right: [w117] -> _
    shift-left: 0 -> [w118]
    tunnel: [w116] -> w14
    tunnel: w11 -> [w115]
    tunnel: w2 -> [w112]
    shift-right: [w111] -> _
    shift-left: _ -> [w110]
    stop <- w120 stop-if-true
    n67 = Dequeue Element(queue=w124, error in (no error)=w115) -> (queue out=w119:refnum<queue>, element=w121:T7, error out=w114:errorcluster)  [unwired: 1 in, 1 out]
    n68 = Equal?(x=w121, y=T7."Quit") -> (x = y?=w120:bool)
    n69 = case shown="\"Init\"" w121 {
      tunnel: w123 -> [w129 w138 w174 w201 w215 w257 w276 w282]
      tunnel: [w129 w138 w186 w200 w223 w262 w275 w282] -> w122
      tunnel: w119 -> [_ w142 w189 w198 w220 w259 w279 _]
      tunnel: w118 -> [w128 w137 _ w202 w210 w256 w274 w281]
      tunnel: [w128 w137 w168 w202 w210 w256 w274 w281] -> w117
      tunnel: [w127 w141 w187 w197 w219 w254 w277 w283] -> w116
      tunnel: w114 -> [w127 w140 w188 w199 w218 w253 w278 w283]
      tunnel: w112 -> [_ w132 _ _ _ _ _ _]
      tunnel: [w126 w136 w175 w195 w209 w252 w273 w280] -> w111
      tunnel: w110 -> [w126 w136 _ w195 w209 w252 w273 w280]
      frame "Idle", Default {
        w125 = FALSE
        n70 = local write "Singleshot Button"(w125) -> ()
        n71 = local write "Loop Button"(w125) -> ()
      }
      frame "Init" {
        w135 = FALSE
        n72 = for {
          N: 8 -> [_]
          tunnel: w132 -> [w144]
          i -> [w145]
          n73 = case shown="0, Standard" w145 {
            tunnel: [w146 w147 w148 w149 w150 w151 w152 w153] -> w143
            frame 0, Default {
              n74 = control-ref of="AI Channel 0"() -> (w146:refnum<vi>)
            }
            frame 1 {
              n75 = control-ref of="AI Channel 1"() -> (w147:refnum<vi>)
            }
            frame 2 {
              n76 = control-ref of="AI Channel 2"() -> (w148:refnum<vi>)
            }
            frame 3 {
              n77 = control-ref of="AI Channel 3"() -> (w149:refnum<vi>)
            }
            frame 4 {
              n78 = control-ref of="AI Channel 4"() -> (w150:refnum<vi>)
            }
            frame 5 {
              n79 = control-ref of="AI Channel 5"() -> (w151:refnum<vi>)
            }
            frame 6 {
              n80 = control-ref of="AI Channel 6"() -> (w152:refnum<vi>)
            }
            frame 7 {
              n81 = control-ref of="AI Channel 7"() -> (w153:refnum<vi>)
            }
          }
          n82 = call "m2p_gui_update_ai_ch.vi"("AI Details"=w144, "Cluster Referenz"=w143, "Channel Index"=w145) -> ()  [unwired: 9 in]
        }
        n83 = control-ref of="Mode Setup"() -> (w134:refnum<vi>)
        n84 = control-ref of="Clock Settings"() -> (w131:refnum<vi>)
        n85 = control-ref of="Trigger Settings"() -> (w130:refnum<vi>)
        n86 = call "gui_update_mode.vi"("Referenz Mode Settings"=w134) -> ()  [unwired: 11 in]
        n87 = call "m2p_gui_update_clock.vi"("Cluster Reference"=w131) -> ()  [unwired: 11 in]
        n88 = call "m2p_gui_update_ai_trig.vi"("Trigger Settings Reference"=w130) -> ()  [unwired: 10 in]
        n89 = local write "Singleshot Button"(w135) -> ()
        n90 = local write "Loop Button"(w135) -> ()
        n91 = local write "Stop Button"(w135) -> ()
        n92 = local write "Force Trigger Button"(w135) -> ()
        n93 = local write "Quit Button"(w135) -> ()
        n94 = Enqueue Element(queue=w142, element=T7."Idle", error in (no error)=w140) -> (error out=w141:errorcluster)  [unwired: 1 in, 2 out]
      }
      frame "Write Setup" {
        w178 = 4096
        # ">> Number of active channels"
        # ">> Bytes per sample"
        # ">> ABA Data Length"
        # "ABA Notify Size"
        # "ABA Buffer Size"
        # "Setup FIFO buffer for ABA data"
        # ">> Number of active channels"
        n95 = call "m2p_setup_ai_channels.vi"("Card Info In"=w174, "AI Channel 4"="AI Channel 4", "AI Channel 5"="AI Channel 5", "AI Channel 0"="AI Channel 0", "AI Channel 1"="AI Channel 1", "AI Channel 2"="AI Channel 2", "AI Channel 3"="AI Channel 3", "AI Channel 6"="AI Channel 6", "AI Channel 7"="AI Channel 7") -> ("Card Info Out"=w173:cluster{"Card Handle":u64, "Error Code":u32}, "ChMask"=w172:i32)  [unwired: 5 in]
        n96 = call "setup mode record standard.vi"("Mode Setup"="Mode Setup", "Channel Mask Low"=w172, "Card Info In"=w173) -> ("Card Info Out"=w171:cluster{"Card Handle":u64, "Error Code":u32})  [unwired: 3 in, 1 out]
        n97 = call "m2p_setup_ai_general.vi"("Card Info In"=w171, "Clock Settings"="Clock Settings", "Trigger Settings"="Trigger Settings") -> ("Card Info Out"=w170:cluster{"Card Handle":u64, "Error Code":u32}, "Used Sampling Rate (kS)"=w167:dbl, "Bytes Per Sample"=w169:i32, "Channel Count"=w168:i32)  [unwired: 9 in]
        n98 = call "dwSetupFIFOMode.vi"("Notify (Bytes)"=w178, "Bufferlength (Bytes)"=40960, "Allocate"=TRUE, "Buffertype (0=data, 1=TS, 2=ABA)"=2, "Card Info In"=w170) -> ("Card Info Out"=w179:cluster{"Card Handle":u64, "Error Code":u32})  [unwired: 4 in]
        n99 = call "error check and message.vi"("Card Info In"=w179) -> ("Error occurred"=w154:bool, "Error Message"=w184:string, "Card Info Out"=w186:cluster{"Card Handle":u64, "Error Code":u32})  [unwired: 4 in]
        n100 = Not(x=w154) -> (.not. x?=w155:bool)
        n101 = case shown="True" w155 {
          tunnel: w167 -> [_ w192]
          frame False {
          }
          frame True {
            # "Write back used sampling rate to clock dialog"
            n102 = local read "Clock Settings"() -> (w191:T2)
            n103 = Bundle By Name(cluster=w191, "Sampling Rate (kHz)"=w192) -> (w190:T2)
            n104 = local write "Clock Settings"(w190) -> ()
          }
        }
        n105 = local write "Status"(w184) -> ()
        n106 = Multiply(x=w168, y=w169) -> (x*y=w177:i32)
        n107 = Divide(x=w178, y=w177) -> (x/y=w176:dbl)
        n108 = case shown="False" w154 {
          tunnel: [T7."Start" T7."Idle"] -> w185
          frame False {
          }
          frame True {
          }
        }
        n109 = To Long Integer(number=w176) -> (32bit integer=w175:i32)
        n110 = Enqueue Element(queue=w189, element=w185, error in (no error)=w188) -> (error out=w187:errorcluster)  [unwired: 1 in, 2 out]
        n111 = local write "Write Setup"(FALSE) -> ()
      }
      frame "Start" {
        n112 = call "cmd start.vi"("Card Info In"=w201) -> ("Card Info Out"=w200:cluster{"Card Handle":u64, "Error Code":u32})  [unwired: 6 in]
        n113 = Enqueue Element(queue=w198, element=T7."Acquire", error in (no error)=w199) -> (error out=w197:errorcluster)  [unwired: 1 in, 2 out]
      }
      frame "Acquire" {
        # ">> ABA Data Length"
        # "Read and plot ABA data"
        n114 = call "read extra status.vi"("Card Info In"=w215) -> ("Overrun"=w212:bool, "Data transfer end"=w207:bool, "Next block ready"=w204:bool, "Card Info Out"=w203:cluster{"Card Handle":u64, "Error Code":u32})  [unwired: 3 in]
        n115 = case shown="True" w212 {
          frame False {
          }
          frame True {
            n116 = One Button Dialog(message="A buffer overrun has occurred. Please check the buffer size and the speed") -> ()  [unwired: 1 in, 1 out]
          }
        }
        n117 = Not(x=w207) -> (.not. x?=w205:bool)
        n118 = And(x=w204, y=w205) -> (x .and. y?=w206:bool)
        n119 = case shown="True" w206 {
          tunnel: w203 -> [w227 w232]
          tunnel: [w227 w231] -> w211
          tunnel: w210 -> [_ w230]
          tunnel: w209 -> [_ w228]
          frame False {
          }
          frame True {
            n120 = call "dwABARead_float.vi"("Card Info In"=w232, "Channel Count"=w230, "Length (Samples per Channel)"=w228) -> ("Card Info Out"=w231:cluster{"Card Handle":u64, "Error Code":u32}, "Ch 0"=w236:sgl[], "Ch 1"=w235:sgl[], "Ch 2"=w234:sgl[], "Ch 3"=w233:sgl[])  [unwired: 8 in, 12 out]
            n121 = Build Array(w236, w235, w234, w233) -> (→"Display ABA Data":sgl[][])
          }
        }
        n122 = call "read card status.vi"("Card Info In"=w211) -> ("Card ready"=w222:bool, "Trigger detected"=w225:bool, "Pretrigger full"=w226:bool, "Card Info Out"=w216:cluster{"Card Handle":u64, "Error Code":u32})  [unwired: 3 in]
        n123 = call "spcm_translate_status.vi"("Ready"=w222, "Trigger"=w225, "Pretrigger"=w226) -> ("Text"=→"Status":string)  [unwired: 4 in]
        n124 = call "error check and message.vi"("Card Info In"=w216) -> ("Error occurred"=w213:bool)  [unwired: 4 in, 2 out]
        n125 = Or(x=w213, y=w212) -> (x .or. y?=w214:bool)
        n126 = Not(x=w214) -> (.not. x?=w217:bool)
        n127 = case shown="True" w217 {
          tunnel: [T11."Quit" w245] -> w224
          tunnel: w222 -> [_ w244]
          frame False {
          }
          frame True {
            n128 = local read "Stop Button"() -> (w239:bool)
            n129 = Select(t=T7."Read Data", s=w244, f=T7."Acquire") -> (s? t:f=w243:T7)
            n130 = Select(t=T7."Stop", s=w239, f=w243) -> (s? t:f=w245:T7)
          }
        }
        n131 = Enqueue Element(queue=w220, element=w224, error in (no error)=w218) -> (error out=w219:errorcluster)  [unwired: 1 in, 2 out]
        n132 = local read "Force Trigger Button"() -> (w208:bool)
        n133 = case shown="True" w208 {
          tunnel: w216 -> [w246 w249]
          tunnel: [w246 w248] -> w223
          frame False {
          }
          frame True {
            n134 = local write "Force Trigger Button"(FALSE) -> ()
            n135 = call "cmd force trigger.vi"("Card Info In"=w249) -> ("Card Info Out"=w248:cluster{"Card Handle":u64, "Error Code":u32})  [unwired: 6 in]
          }
        }
      }
      frame "Read Data" {
        # ">> Number of active channels"
        n136 = local read "Mode Setup"() -> (w250:T5)
        n137 = Unbundle By Name(w250) -> ("Mem"=w258:u32)
        n138 = local read "Loop Button"() -> (w251:bool)
        n139 = call "dwDataRead_float.vi"("Card Info In"=w257, "Channel Count"=w256, "Length (Samples per Channel)"=w258) -> ("Card Info Out"=w262:cluster{"Card Handle":u64, "Error Code":u32}, "Ch 0"=w265:sgl[], "Ch 1"=w264:sgl[], "Ch 2"=w263:sgl[], "Ch 3"=w261:sgl[])  [unwired: 8 in, 12 out]
        n140 = Build Array(w265, w264, w263, w261) -> (→"Display Data":sgl[][])
        n141 = case shown="True" w251 {
          tunnel: [T11."Idle" w270] -> w255
          frame False {
          }
          frame True {
            n142 = local read "Write Setup"() -> (w267:bool)
            n143 = Select(t=T7."Write Setup", s=w267, f=T7."Start") -> (s? t:f=w270:T7)
          }
        }
        n144 = Enqueue Element(queue=w259, element=w255, error in (no error)=w253) -> (error out=w254:errorcluster)  [unwired: 1 in, 2 out]
      }
      frame "Stop" {
        n145 = call "cmd stop.vi"("Card Info In"=w276) -> ("Card Info Out"=w275:cluster{"Card Handle":u64, "Error Code":u32})  [unwired: 6 in]
        n146 = Enqueue Element(queue=w279, element=T7."Idle", error in (no error)=w278) -> (error out=w277:errorcluster)  [unwired: 1 in, 2 out]
        n147 = local write "Status"("Stopped") -> ()
      }
      frame "Quit" {
      }
    }
  }
  n148 = Merge Errors(w15, w14) -> (w13:errorcluster)
  n149 = Release Queue(queue=w12, error in (no error)=w13) -> ()  [unwired: 1 in, 3 out]
  n150 = call "spcm_vClose.vi"("Card Info In"=w26) -> ()  [unwired: 7 in]
